vi "led.vi"() -> ()   [LabVIEW 2011]
uses:
  <vilib>/LabVIEW Interface for Arduino/Type Defs/Pin Mode.ctl
  <vilib>/LabVIEW Interface for Arduino/Type Defs/Board Type.ctl
  <vilib>/LabVIEW Interface for Arduino/Type Defs/Connection Type.ctl
  <vilib>/LabVIEW Interface for Arduino/LabVIEW Interface for Arduino.lvlib
panel:
  in  "Baud Rate (115200)":u32=115200
  in  "Connection Type (USB/Serial)":T1
  in  "?":T2
  in  "?":refnum<visa-resource-name>
  in  "LED Status":bool
  in  "Pin Mode (Input)":T3
  in  "Digital I/O Pin":u8
  in  "stop":bool
  # "Ulisesgascon.com"
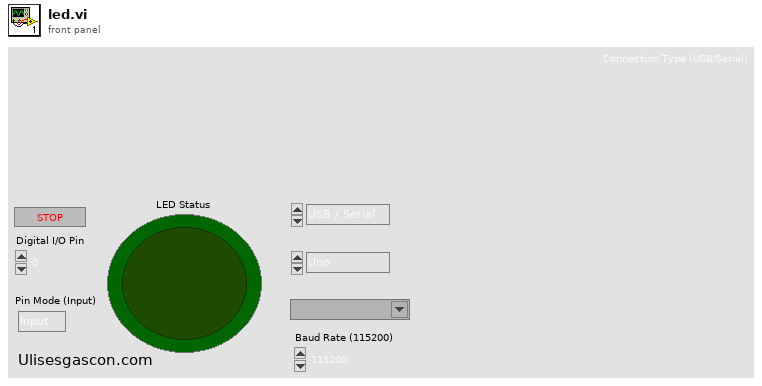
[diagram p1: front panel]
types:
  T1 = typedef "LabVIEW Interface for Arduino.lvlib/Connection Type.ctl" = enum8{"USB / Serial", "XBEE", "BlueSmirf (Bluetooth)"}
  T2 = typedef "LabVIEW Interface for Arduino.lvlib/Board Type.ctl" = enum16{"Uno", "Dimuelanove w/Atmega 328", "Mega 2560"}
  T3 = typedef "LabVIEW Interface for Arduino.lvlib/Pin Mode.ctl" = enum8{"Input", "Output"}
  T4 = typedef "LabVIEW Interface for Arduino.lvlib/Arduino Resource.ctl" = cluster{"VISA resource":refnum<visa-resource-name>, "Board Type":T2, "Connection Type":enum8{"USB / Serial"}, "Bytes Per Packet (15)":u8}
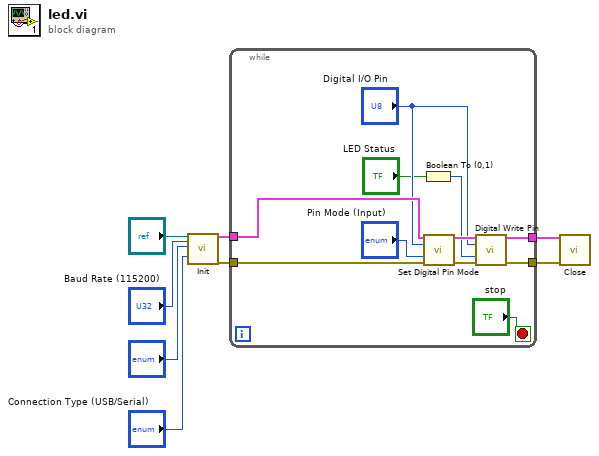
[diagram p0: block diagram]
diagram:
  n1 = call <vilib>:"Init.vi"("VISA resource"="?", "Baud Rate (115200)"="Baud Rate (115200)", "Board Type (Uno)"="?", "Connection Type (USB/Serial)"="Connection Type (USB/Serial)") -> ("Arduino Resource"=w8:T4, "error out"=w7:errorcluster)  [unwired: 14 in]
  n2 = while {
    tunnel: w8 -> [w18]
    tunnel: w7 -> [w17]
    tunnel: [w14] -> w6
    tunnel: [w13] -> w5
    stop <- "stop" stop-if-true
    n3 = Boolean To (0,1)(Boolean="LED Status") -> (0, 1=w10:i16)
    n4 = call <vilib>:"Set Digital Pin Mode.vi"("Arduino Resource"=w18, "Digital I/O Pin"="Digital I/O Pin", "Pin Mode (Input)"="Pin Mode (Input)", "error in"=w17) -> ("Arduino Resource"=w15:T4, "error out"=w16:errorcluster)  [unwired: 10 in]
    n5 = call <vilib>:"Digital Write Pin.vi"("Arduino Resource"=w15, "Digital I/O Pin (0)"="Digital I/O Pin", "Value (0)"=w10, "error in"=w16) -> ("Arduino Resource"=w14:T4, "error out"=w13:errorcluster)  [unwired: 10 in]
  }
  n6 = call <vilib>:"Close.vi"("Arduino Resource"=w6, "error in"=w5) -> ()  [unwired: 13 in, 1 out]
